vi "GenerateFilenames.vi"(11 "Path":path) -> (3 "Array":string[](array[string]))   [LabVIEW 2019]
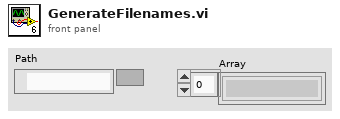
[diagram p1: front panel]
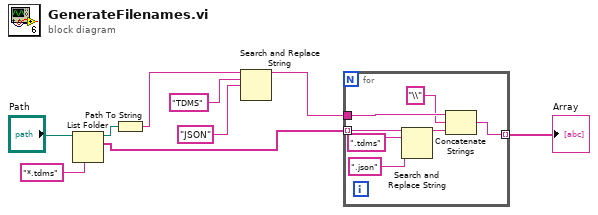
[diagram p0: block diagram]
diagram:
  n1 = List Folder(path="Path", pattern="*.tdms") -> (path out=w7:path, filenames=w9:string[])  [unwired: 2 in, 2 out]
  n2 = Path To String(path=w7) -> (string=w8:string)
  n3 = Search and Replace String(input string=w8, search string="TDMS" ("input string"), replace string="JSON" ("replace string (\"\")")) -> (result string=w4:string)  [unwired: 5 in, 3 out]
  n4 = for {
    tunnel: w9 -> [w12] mode=indexing
    tunnel: [w16] -> w5 mode=indexing
    tunnel: w4 -> [w15]
    n5 = Search and Replace String(input string=w12, search string=".tdms", replace string=".json" ("replace string (\"\")")) -> (result string=w13:string)  [unwired: 5 in, 3 out]
    n6 = Concatenate Strings(w15, "\\" ("string"), w13) -> (w16:string)
  }
  "Array" <- w5
